vi "TstBldr_InitVS_Sequence.vi"(8 "error in":errorcluster, 9 "VeriStand version info":T1, 10 "Sequence File Ref":refnum<k7>, 11 "Engine Reference":refnum<k7>) -> (0 "error out":errorcluster, 1 "VeriStand version info (out)":T1, 2 "Sequence File Ref(out)":refnum<k7>, 3 "Engine reference(out)":refnum<k7>)   [LabVIEW 2011]
doc: "This VI creates the necessary object references in TestStand and adds the steps to open VeriStand managers' references"
uses:
  SeqBuilder/Ctls/dotNetAssemblyInfo.ctl
  SeqBuilder/Ctls/VSModuleTokens.ctl
  VS_InitSteps.ctl
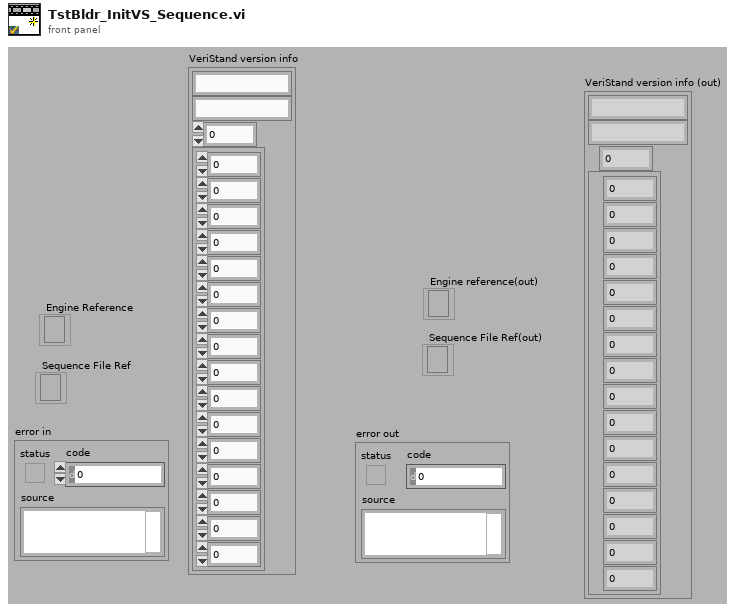
[diagram p1: front panel]
types:
  T1 = typedef "dotNetAssemblyInfo.ctl" = cluster{"VeriStand.exe Path":string, "Assembly":string, "Constructor Token":i32, "Module Token":T2}
  T2 = typedef "VSModuleTokens.ctl" = cluster{"GetIWorkspaceToken":i32, "GetIStimulusToken":i32, "GetIModelManagerToken":i32, "GetIProjectToken":i32, "RunProjectToken":i32, "CloseProjectToken":i32, "RunWorkspaceToken":i32, "StopWorkspaceToken":i32, "SetSingleChannelToken":i32, "SetMultipleParametersToken":i32, "RunStimulusToken":i32, "GetStimulusStateToken":i32, "Open WorkspaceToken":i32, "DeployToken":i32, "UndeployToken":i32, "QuitToken":i32}
  T3 = typedef "VS_InitSteps.ctl" = enum16{"Call VeriStand", "Open Interface", "Do While", "Open Workspace Ref", "Wait", "End", "Open Stim Profile Mngr Ref", "Open Model Mngr Ref", "Quit VeriStand"}
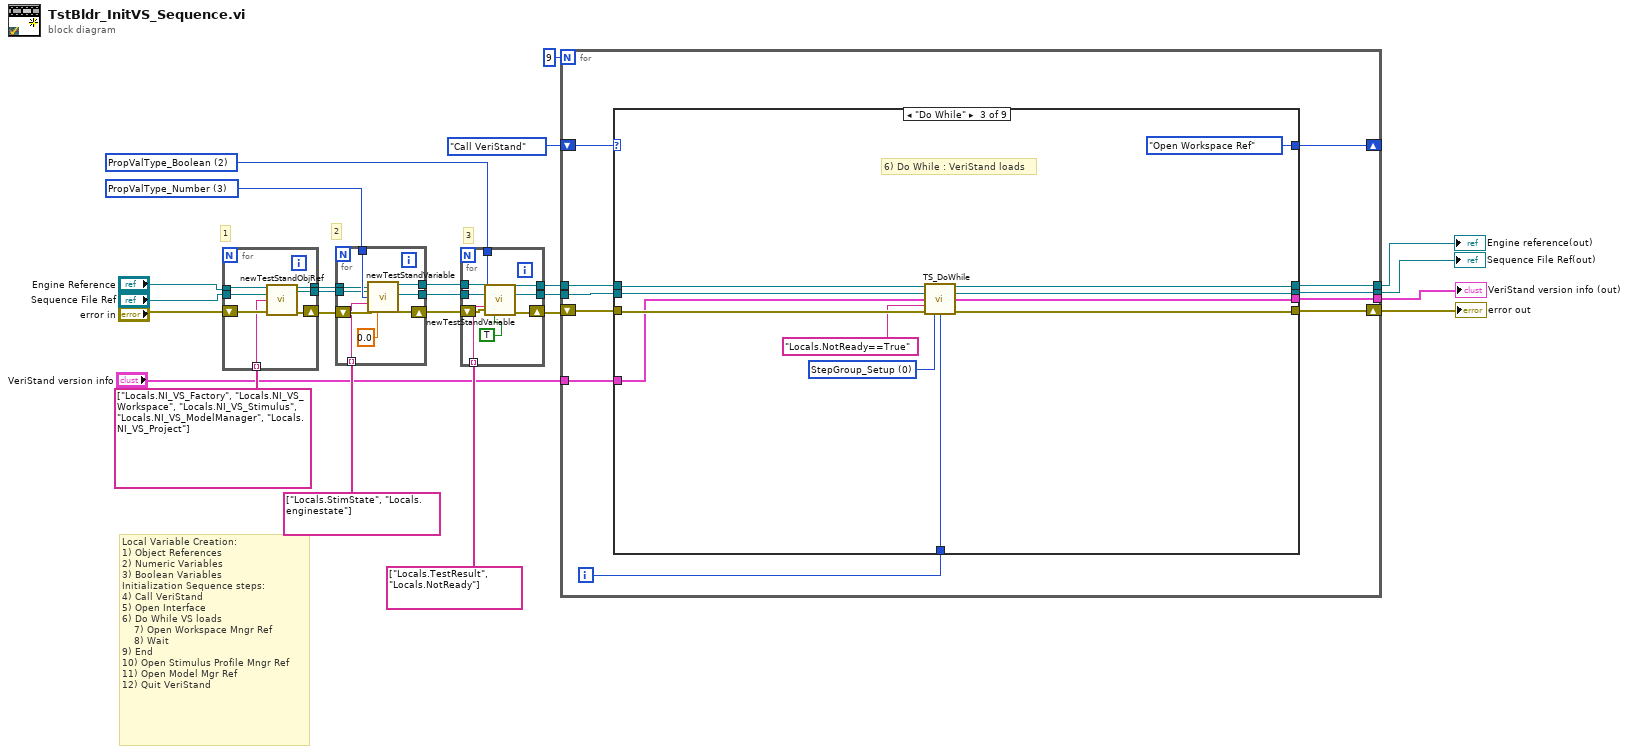
[diagram p0: block diagram]
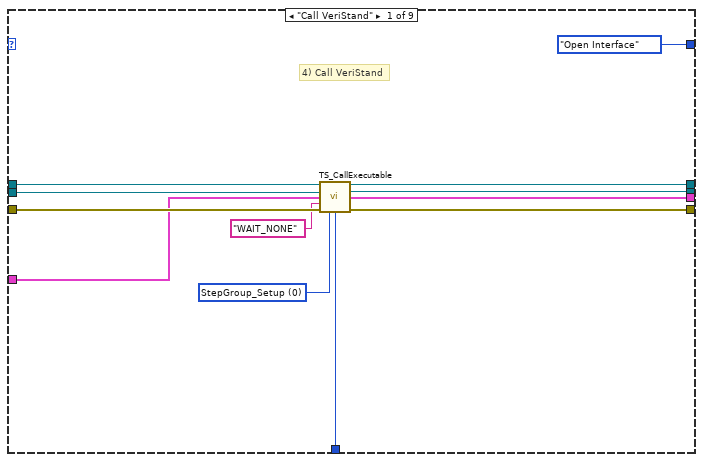
[diagram p2: hidden frame]
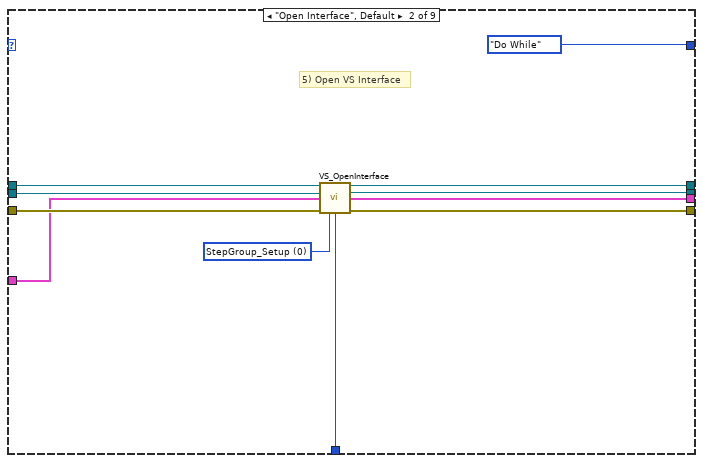
[diagram p3: hidden frame]
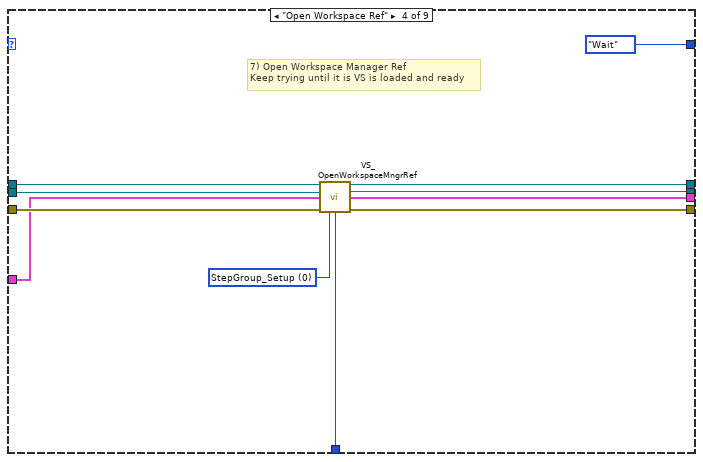
[diagram p4: hidden frame]
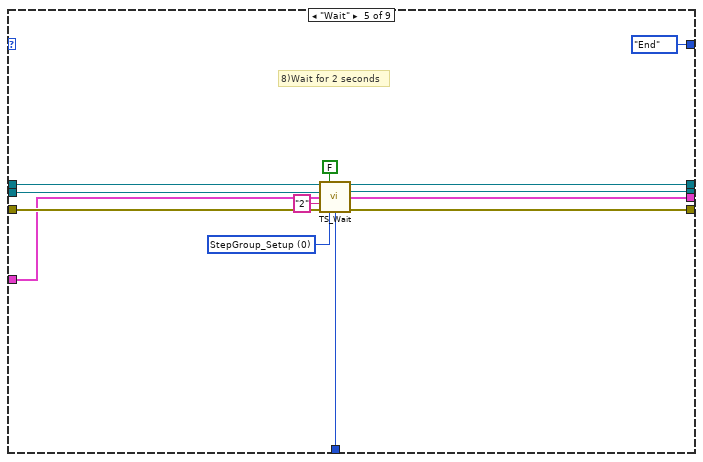
[diagram p5: hidden frame]
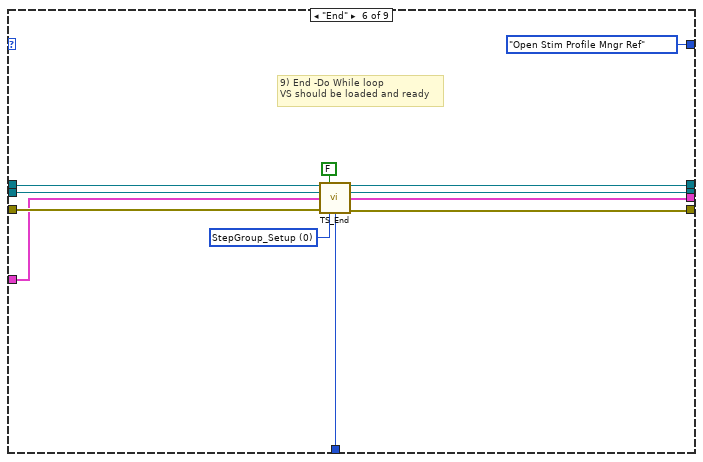
[diagram p6: hidden frame]
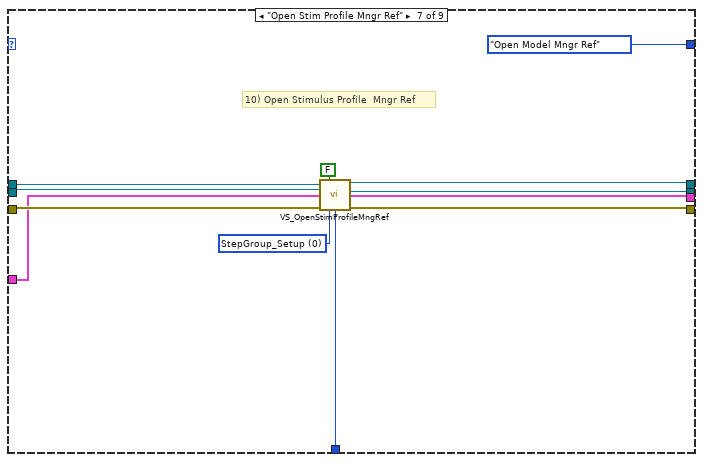
[diagram p7: hidden frame]
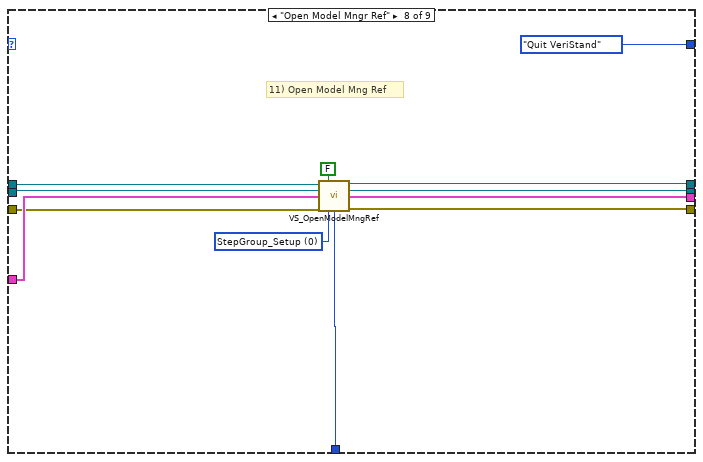
[diagram p8: hidden frame]
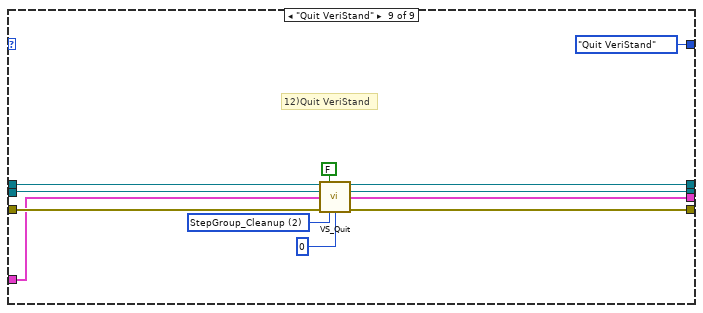
[diagram p9: hidden frame]
diagram:
  w6 = 3 items=["PropValType_Container", "PropValType_String", "PropValType_Boolean", "PropValType_Number", "PropValType_NamedType", "PropValType_Reference", "PropValType_Array"] ("Variable Type")
  w11 = 2 items=["PropValType_Container", "PropValType_String", "PropValType_Boolean", "PropValType_Number", "PropValType_NamedType", "PropValType_Reference", "PropValType_Array"] ("Variable Type")
  # "Local Variable Creation:\n1) Object References\n2) Numeric Variables\n3) Boolean Variables\nInitialization Sequence steps:\n4) Call VeriStand\n5) Open Interface\n6) Do While VS loads\n    7) Open Workspace Mngr Ref\n    8) Wait\n9) End\n10) Open Stimulus Profile Mngr Ref\n11) Open Model Mgr Ref\n12) Quit VeriStand"
  # "3"
  # "2"
  # "1"
  n1 = for {
    tunnel: "Engine Reference" -> [w28]
    tunnel: "Sequence File Ref" -> [w27]
    tunnel: string[] ["Locals.NI_VS_Factory", "Locals.NI_VS_Workspace", "Locals.NI_VS_Stimulus", "Locals.NI_VS_ModelManager", "Locals.NI_VS_Project"] -> [w25] mode=indexing
    tunnel: [w30] -> w4
    tunnel: [w29] -> w3
    shift-right: [w31] -> w5
    shift-left: "error in" -> [w26]
    n2 = call "newTestStandObjRef.vi"("Engine Reference"=w28, "Sequence File Ref"=w27, "Variable Name"=w25, "error in"=w26) -> ("Engine Reference (out)"=w30:refnum<k7>, "Sequence File (out)"=w29:refnum<k7>, "error out"=w31:errorcluster)  [unwired: 9 in]
  }
  n3 = for {
    tunnel: string[] ["Locals.StimState", "Locals.enginestate"] -> [w33] mode=indexing
    tunnel: [w40] -> w9
    tunnel: [w39] -> w8
    tunnel: w6 -> [w37]
    tunnel: w4 -> [w35]
    tunnel: w3 -> [w34]
    shift-right: [w38] -> w7
    shift-left: w5 -> [w36]
    n4 = call "newTestStandVariable.vi"("Engine Reference"=w35, "Sequence File Ref"=w34, "Variable Type"=w37, "Variable Name"=w33, "error in"=w36, "Variable Value"=0.0) -> ("Engine Reference(out)"=w40:refnum<k7>, "Sequence File Ref(out)"=w39:refnum<k7>, "error out"=w38:errorcluster)  [unwired: 7 in]
  }
  n5 = for {
    tunnel: [w48] -> w13
    tunnel: [w47] -> w12
    tunnel: w11 -> [w46]
    tunnel: string[] ["Locals.TestResult", "Locals.NotReady"] -> [w45] mode=indexing
    tunnel: w9 -> [w44]
    tunnel: w8 -> [w43]
    shift-right: [w49] -> w14
    shift-left: w7 -> [w42]
    n6 = call "newTestStandVariable.vi"("Engine Reference"=w44, "Sequence File Ref"=w43, "Variable Type"=w46, "Variable Name"=w45, "error in"=w42, "Variable Value"=TRUE) -> ("Engine Reference(out)"=w47:refnum<k7>, "Sequence File Ref(out)"=w48:refnum<k7>, "error out"=w49:errorcluster)  [unwired: 7 in]
  }
  n7 = for {
    N: 9 -> [_]
    tunnel: w12 -> [w59]
    tunnel: w13 -> [w57]
    tunnel: [w56] -> w20
    shift-right: [w55] -> w21
    shift-left: w14 -> [w58]
    shift-right: [w53] -> _
    shift-left: VS_InitSteps."Call VeriStand" ("Enum") -> [w60]
    tunnel: [w52] -> w22
    tunnel: "VeriStand version info" -> [w51]
    tunnel: [w50] -> w1
    i -> [w54]
    n8 = case shown="\"Do While\"" w60 {
      tunnel: w59 -> [w70 w83 w95 w105 w117 w131 w141 w154 w166]
      tunnel: w58 -> [w71 w82 w93 w103 w119 w129 w142 w150 w165]
      tunnel: w57 -> [w69 w81 w94 w104 w118 w126 w140 w152 w164]
      tunnel: [w66 w76 w90 w100 w115 w127 w137 w147 w161] -> w56
      tunnel: [w67 w77 w89 w102 w114 w128 w136 w146 w160] -> w55
      tunnel: w54 -> [w64 w78 w88 w98 w113 w123 w135 w149 _]
      tunnel: [VS_InitSteps."Open Interface" ("Enum") VS_InitSteps."Do While" VS_InitSteps."Open Workspace Ref" VS_InitSteps."Wait" VS_InitSteps."End" VS_InitSteps."Open Stim Profile Mngr Ref" VS_InitSteps."Open Model Mngr Ref" VS_InitSteps."Quit VeriStand" VS_InitSteps."Quit VeriStand"] -> w53
      tunnel: [w65 w75 w91 w101 w116 w130 w138 w153 w162] -> w52
      tunnel: w51 -> [w63 w79 w92 w99 w111 w125 w139 w151 w163]
      tunnel: [w62 w74 w84 w97 w107 w120 w132 w144 w156] -> w50
      frame "Call VeriStand" {
        w61 = 0 items=["StepGroup_Setup", "StepGroup_Main", "StepGroup_Cleanup"] ("Step Group")
        # "4) Call VeriStand"
        n9 = call "TS_CallExecutable.vi"("Engine Reference(in)"=w70, "Sequence File Ref(in)"=w69, "VeriStand version info"=w63, "Wait Condition"="WAIT_NONE", "error in"=w71, "Step Group"=w61, "index"=w64) -> ("Engine reference(out)"=w65:refnum<k7>, "Sequence File Ref(out)"=w66:refnum<k7>, "VeriStand verion info(out)"=w62:T1, "error out"=w67:errorcluster)  [unwired: 5 in]
      }
      frame "Open Interface", Default {
        w73 = 0 items=["StepGroup_Setup", "StepGroup_Main", "StepGroup_Cleanup"] ("Step Group")
        # "5) Open VS Interface"
        n10 = call "VS_OpenInterface.vi"("Engine Reference(in)"=w83, "Sequence File Ref(in)"=w81, "VeriStand version info"=w79, "error in"=w82, "Step Group"=w73, "Step Index"=w78) -> ("Engine reference(out)"=w75:refnum<k7>, "Sequence File Ref(out)"=w76:refnum<k7>, "VeriStand version info (out)"=w74:T1, "error out"=w77:errorcluster)  [unwired: 6 in]
      }
      frame "Do While" {
        w87 = 0 items=["StepGroup_Setup", "StepGroup_Main", "StepGroup_Cleanup"] ("Step Group")
        # "6) Do While : VeriStand loads"
        n11 = call "TS_DoWhile.vi"("Engine Reference(in)"=w95, "Sequence File Ref(in)"=w94, "VeriStand version info"=w92, "Condition"="Locals.NotReady==True", "error in"=w93, "Step Group"=w87, "index"=w88) -> ("Engine reference(out)"=w91:refnum<k7>, "Sequence File Ref(out)"=w90:refnum<k7>, "VeriStand verion info(out)"=w84:T1, "error out"=w89:errorcluster)  [unwired: 5 in]
      }
      frame "Open Workspace Ref" {
        w96 = 0 items=["StepGroup_Setup", "StepGroup_Main", "StepGroup_Cleanup"] ("Step Group")
        # "7) Open Workspace Manager Ref\nKeep trying until it is VS is loaded and ready"
        n12 = call "VS_OpenWorkspaceMngrRef.vi"("Engine Reference(in)"=w105, "Sequence File Ref(in)"=w104, "VeriStand version info"=w99, "error in"=w103, "Step Group"=w96, "Step Index"=w98) -> ("Engine reference(out)"=w101:refnum<k7>, "Sequence File Ref(out)"=w100:refnum<k7>, "VeriStand version info (out)"=w97:T1, "error out"=w102:errorcluster)  [unwired: 6 in]
      }
      frame "Wait" {
        w112 = 0 items=["StepGroup_Setup", "StepGroup_Main", "StepGroup_Cleanup"] ("Step Group")
        # "8)Wait for 2 seconds"
        n13 = call "TS_Wait.vi"("Engine Reference(in)"=w117, "Condition Run?"=FALSE, "Sequence File Ref(in)"=w118, "VeriStand version info"=w111, "Time to Wait"="2", "error in"=w119, "Step Group"=w112, "index"=w113) -> ("Engine reference(out)"=w116:refnum<k7>, "Sequence File Ref(out)"=w115:refnum<k7>, "VeriStand verion info(out)"=w107:T1, "error out"=w114:errorcluster)  [unwired: 4 in]
      }
      frame "End" {
        w122 = 0 items=["StepGroup_Setup", "StepGroup_Main", "StepGroup_Cleanup"] ("Step Group")
        # "9) End -Do While loop\nVS should be loaded and ready"
        n14 = call "TS_End.vi"("Engine Reference(in)"=w131, "Condition Run?"=FALSE, "Sequence File Ref(in)"=w126, "VeriStand version info"=w125, "error in"=w129, "Step Group"=w122, "index"=w123) -> ("Engine reference(out)"=w130:refnum<k7>, "Sequence File Ref(out)"=w127:refnum<k7>, "VeriStand verion info(out)"=w120:T1, "error out"=w128:errorcluster)  [unwired: 5 in]
      }
      frame "Open Stim Profile Mngr Ref" {
        w134 = 0 items=["StepGroup_Setup", "StepGroup_Main", "StepGroup_Cleanup"] ("Step Group")
        # "10) Open Stimulus Profile  Mngr Ref"
        n15 = call "VS_OpenStimProfileMngRef.vi"("Engine Reference(in)"=w141, "Condition Run?"=FALSE, "Sequence File Ref(in)"=w140, "VeriStand version info"=w139, "error in"=w142, "Step Group"=w134, "Step Index"=w135) -> ("Engine reference(out)"=w138:refnum<k7>, "Sequence File Ref(out)"=w137:refnum<k7>, "VeriStand version info (out)"=w132:T1, "error out"=w136:errorcluster)  [unwired: 5 in]
      }
      frame "Open Model Mngr Ref" {
        w148 = 0 items=["StepGroup_Setup", "StepGroup_Main", "StepGroup_Cleanup"] ("Step Group")
        # "11) Open Model Mng Ref"
        n16 = call "VS_OpenModelMngRef.vi"("Engine Reference(in)"=w154, "Condition Run?"=FALSE, "Sequence File Ref(in)"=w152, "VeriStand version info"=w151, "error in"=w150, "Step Group"=w148, "Step Index"=w149) -> ("Engine reference(out)"=w153:refnum<k7>, "Sequence File Ref(out)"=w147:refnum<k7>, "VeriStand version info (out)"=w144:T1, "error out"=w146:errorcluster)  [unwired: 5 in]
      }
      frame "Quit VeriStand" {
        w159 = 2 items=["StepGroup_Setup", "StepGroup_Main", "StepGroup_Cleanup"] ("Step Group")
        # "12)Quit VeriStand"
        n17 = call "VS_Quit.vi"("Engine Reference(in)"=w166, "Condition Run?"=FALSE, "Sequence File Ref(in)"=w164, "VeriStand version info"=w163, "error in"=w165, "Step Group"=w159, "Step Index"=0) -> ("Engine reference(out)"=w162:refnum<k7>, "Sequence File Ref(out)"=w161:refnum<k7>, "VeriStand version info (out)"=w156:T1, "error out"=w160:errorcluster)  [unwired: 5 in]
      }
    }
  }
  "error out" <- w21
  "Engine reference(out)" <- w22
  "Sequence File Ref(out)" <- w20
  "VeriStand version info (out)" <- w1
